vi "RunTimeObjectsSectionUI.vi"() -> ()   [LabVIEW 2019, in "RunTimeObjectsSection.lvclass"]
uses:
  RunTimeObjectsSection.lvclass
  <vilib>/NI/Configuration Framework/Node/NodeRef.ctl
  <vilib>/NI/Configuration Framework/Node/NISE_CEF_Node.lvclass
  <vilib>/NI/AMC/Message Queue.ctl
  <vilib>/NI/AMC/Message.ctl
  <vilib>/NI/Tools/Keyed Array/KeyedArray.ctl
  <vilib>/NI/Configuration Framework/Node/UserEventRef.ctl
  <vilib>/NI/Configuration Framework/Controls/EventCluster.ctl
  <vilib>/Utility/sysdir.llb/System Directory Type.ctl
  Controls/RunTimeObjectTypes.ctl
  RunTimeObjectsSection.lvclass/RunTimeObjectsSection.ctl
  Read RunTimeObjectType.vi
  subVI/Global Settings.vi
  Configuration Tool.lvlib
  <vilib>/NI/Tools/Keyed Array/Tools_KeyedArray.lvlib
  <vilib>/NI/AMC/AMC.lvlib
  <vilib>/NI/Configuration Framework/NISE_CEF_TreeControl.lvlib
panel:
  in  "Main UI Tab":enum32{"Page Group"}(tab)
  in  "WebBrowser":refnum<k7>(container)
  in  "user event":T1
  in  "main queue":T2
  in  "node ref":T3
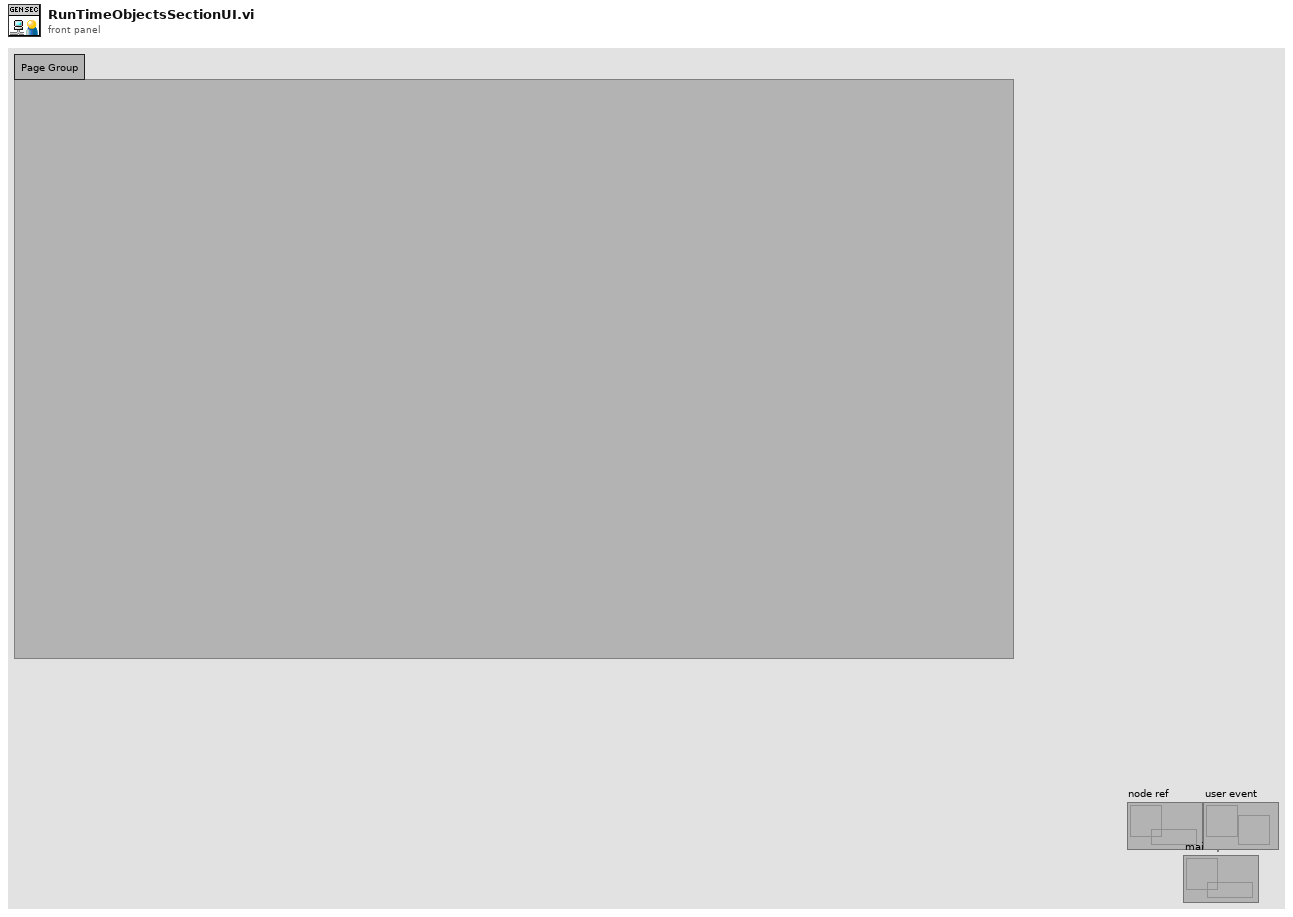
[diagram p1: front panel]
types:
  T1 = typedef "NISE_CEF_Node.lvclass/UserEventRef.ctl" = refnum<user-event>
  T2 = typedef "AMC.lvlib/Message Queue.ctl" = refnum<queue>
  T3 = typedef "NISE_CEF_Node.lvclass/NodeRef.ctl" = refnum<data-value>
  T4 = typedef "Configuration Tool.lvlib/RunTimeObjectTypes.ctl" = enum16{"ActionVIs", "ButtonList", "RunTimeMenu"}
  T5 = typedef "System Directory Type.ctl" = i32
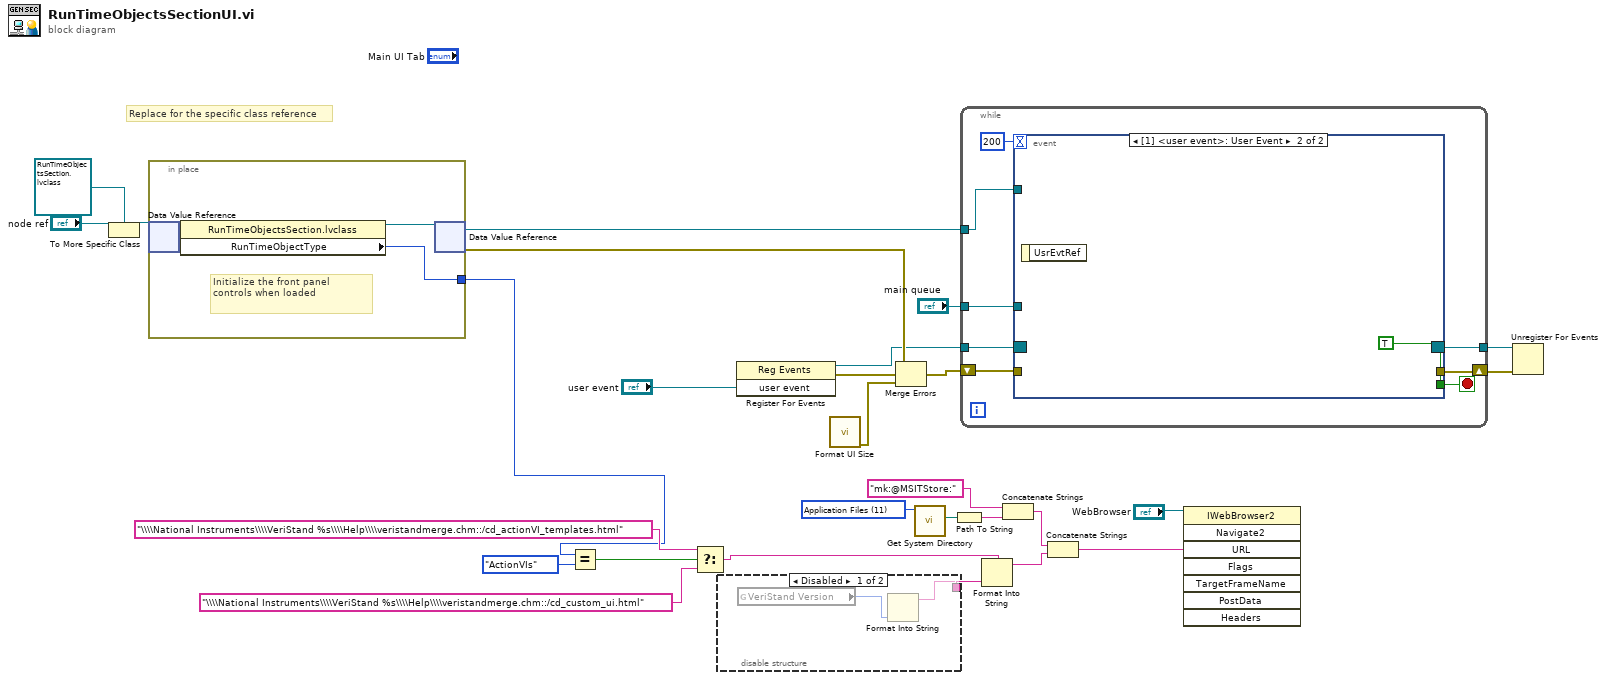
[diagram p0: block diagram]
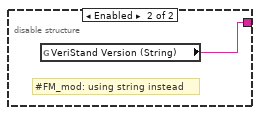
[diagram p2: hidden frame]
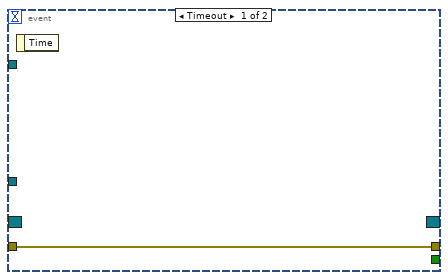
[diagram p3: hidden frame]
diagram:
  w28 = T5 11 items=["User Home"=0, "User Desktop"=1, "User Documents"=2, "User Application Data"=3, "User Preferences"=4, "User Temporary"=5, "Public Documents"=6, "Public Application Data"=7, "Public Preferences"=8, "Public Cache"=13, "System Core Libraries"=9, "System Installed Libraries"=10, "Application Files"=11, "Boot Volume Root"=12] ("system directory type")
  # "Replace for the specific class reference"
  n1 = To More Specific Class(target class=refnum<data-value> refnum ("data value reference"), reference="node ref") -> (specific class reference=w19:refnum<data-value>)  [unwired: 1 in, 1 out]
  n2 = in-place {
    in-place-border: [w29] -> w10
    # "Initialize the front panel controls when loaded"
    n3 = in-place-dvr #1(w19) -> (w31:refnum<class "RunTimeObjectsSection.lvclass">)  [unwired: 1 out]
    n4 = property class="RunTimeObjectsSection.lvclass"(reference=w31) -> (reference out=w30:refnum<class "RunTimeObjectsSection.lvclass">, "RunTimeObjectType"=w29:T4)  [unwired: 1 in, 1 out]
    n5 = in-place-dvr #1(w30) -> (w21:refnum<data-value>, w17:errorcluster)
  }
  n6 = Equal?(x=w10, y=RunTimeObjectTypes."ActionVIs") -> (x = y?=w14:bool)
  n7 = Select(t="\\\\National Instruments\\\\VeriStand %s\\\\Help\\\\veristandmerge.chm::/cd_actionVI_templates.html", s=w14, f="\\\\National Instruments\\\\VeriStand %s\\\\Help\\\\veristandmerge.chm::/cd_custom_ui.html") -> (s? t:f=w12:string)
  n8 = disable-structure shown="Disabled" {
    disable-tunnel: [w32 w34] -> w1
    frame Disabled {
      n9 = global read "Global Settings.vi" "VeriStand Version"() -> (w33:enum16{"2013", "2014", "2015", "2016"})
      n10 = Format Into String(w33) -> (resulting string=w32:string)  [unwired: 3 in, 1 out]
    }
    frame Enabled {
      # "#FM_mod: using string instead"
      n11 = global read "Global Settings.vi" "VeriStand Version (String)"() -> (w34:string)
    }
  }
  n12 = register-events("user event") -> (reference out=w7:refnum<event-registration>, error out=w4:errorcluster)  [unwired: 2 in]
  n13 = call "Format UI Size.vi"() -> ("error out"=w2:errorcluster)  [unwired: 11 in]
  n14 = Merge Errors(w17, w4, w2) -> (w3:errorcluster)
  n15 = call <vilib>:"Get System Directory.vi"("system directory type"=w28) -> ("system directory"=w27:path)  [unwired: 10 in]
  n16 = Path To String(path=w27) -> (string=w26:string)
  n17 = while {
    tunnel: w21 -> [w42]
    tunnel: "main queue" -> [w41]
    tunnel: w7 -> [w39]
    tunnel: [w38] -> w6
    shift-right: [w36] -> w5
    shift-left: w3 -> [w35]
    stop <- w37 stop-if-true
    n18 = event shown="[1] <user event>: User Event" {
      selector: w39 -> [_ _]
      dyn-events: [_ _] -> w38
      timeout: 200 -> [_ _]
      tunnel: w42 -> [_ _]
      tunnel: w41 -> [_ _]
      tunnel: [_ TRUE] -> w37
      tunnel: [w43 _] -> w36
      tunnel: w35 -> [w43 _]
      event Timeout {
        n19 = event-data() -> ()  [unwired: 1 in, 1 out]
      }
      event User Event {
        n20 = event-data() -> ()  [unwired: 1 in, 1 out]
      }
    }
  }
  n21 = Format Into String(format string=w12, w1) -> (resulting string=w23:string)  [unwired: 2 in, 1 out]
  n22 = Concatenate Strings("mk:@MSITStore:" ("concatenated string"), w26) -> (w24:string)
  n23 = Concatenate Strings(w24, w23) -> (w11:string)
  n24 = invoke class="IWebBrowser2" method="Navigate2"(reference="WebBrowser", "URL"=w11) -> ()  [unwired: 6 in, 8 out]
  n25 = Unregister For Events(event registration refnum=w6, error in=w5) -> ()  [unwired: 1 out]
